vi "Bezier curve.vi"(2 "Segments":dbl, 3 "Parameters":cluster{"X":dbl, "Y":dbl}[](array[cluster])) -> (0 "XY Graph":cluster{dbl[], dbl[]}[](graph), 1 "Coordinate Array":cluster{"X":dbl, "Y":dbl}[](array[cluster]))   [LabVIEW 2020]
doc: "This VI uses the equation for a Bézier curve to create a set of coordinates."
panel:
  # "Test the Bezier curves"
  # "Formula:    B(t)  =  (1-t)^3 * P0 + 3 * (1-t)^2 * t * P1 + 3 * (1-t) * t^2 * P2 + t^3 * P3"
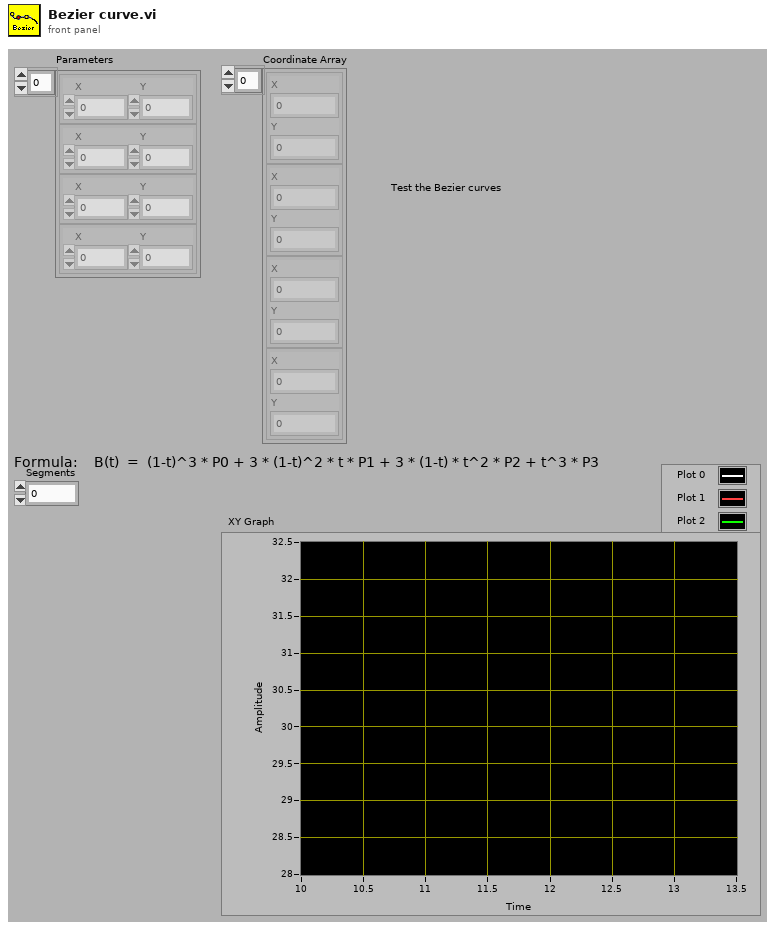
[diagram p1: front panel]
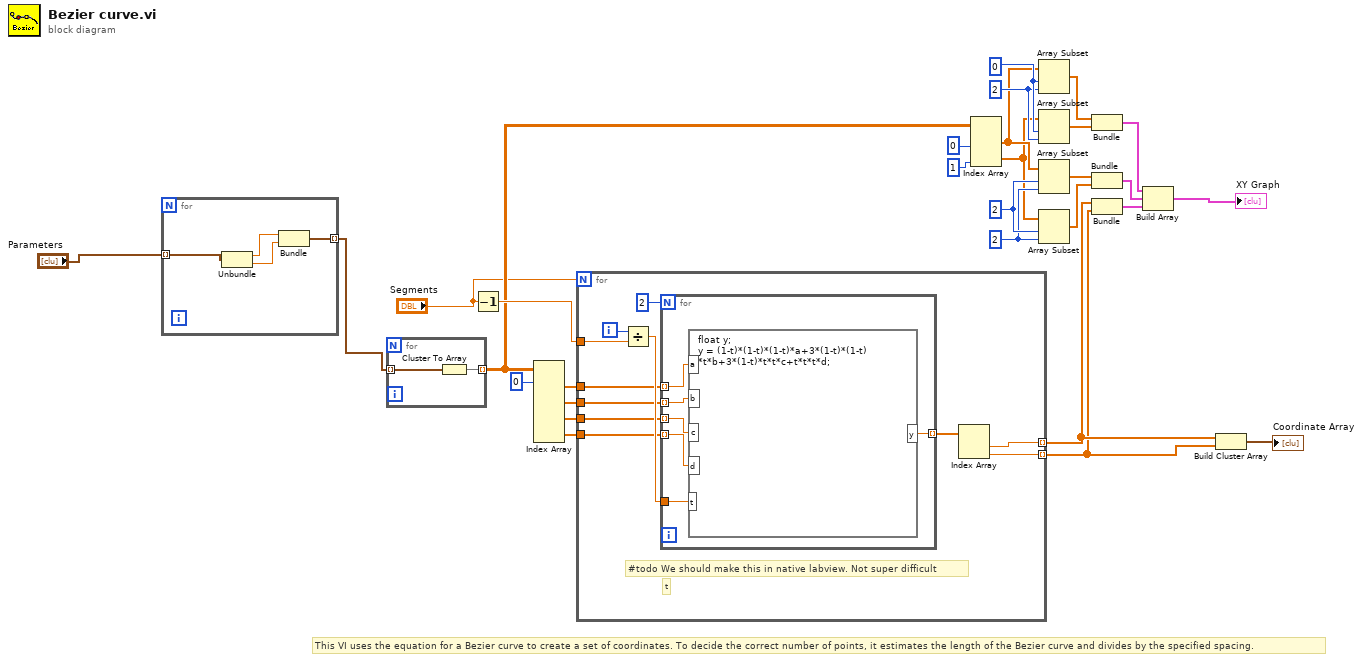
[diagram p0: block diagram]
diagram:
  w24 = 2 ("length")
  w25 = 2 ("index")
  w26 = 2 ("length")
  w27 = 0 ("index")
  # "This VI uses the equation for a Bezier curve to create a set of coordinates. To decide the correct number of points, it estimates the length of the Bezier curve and divides by the specified spacing."
  n1 = for {
    tunnel: "Parameters" -> [w33] mode=indexing
    tunnel: [w31] -> w3 mode=indexing
    n2 = Unbundle(w33) -> ("X"=w32:dbl, "Y"=w30:dbl)
    n3 = Bundle("X"=w32, "Y"=w30) -> (w31:cluster{"X":dbl, "Y":dbl})  [unwired: 1 in]
  }
  n4 = for {
    tunnel: w3 -> [w35] mode=indexing
    tunnel: [w34] -> w5 mode=indexing
    n5 = Cluster To Array(cluster=w35) -> (array=w34:dbl[])
  }
  n6 = Decrement(x="Segments") -> (x-1=w14:dbl)
  n7 = Index Array(array=w5, index (row) #1=0 ("index (row)")) -> (element #1=w12:dbl[], element #2=w11:dbl[], element #3=w10:dbl[], element #4=w9:dbl[])  [unwired: 7 in]
  n8 = for {
    N: "Segments" -> [_]
    tunnel: w12 -> [w43]
    tunnel: w14 -> [w45]
    tunnel: w11 -> [w42]
    tunnel: w10 -> [w41]
    tunnel: w9 -> [w40]
    tunnel: [w38] -> w7 mode=indexing
    tunnel: [w37] -> w2 mode=indexing
    i -> [w46]
    # "#todo We should make this in native labview. Not super difficult"
    # "t"
    n9 = Divide(x=w46, y=w45) -> (x/y=w44:dbl)
    n10 = for {
      N: 2 -> [_]
      tunnel: w44 -> [w52]
      tunnel: w43 -> [w51] mode=indexing
      tunnel: w42 -> [w50] mode=indexing
      tunnel: w41 -> [w49] mode=indexing
      tunnel: w40 -> [w48] mode=indexing
      tunnel: [w47] -> w39 mode=indexing
      n11 = formula code="float y;\ny = (1-t)*(1-t)*(1-t)*a+3*(1-t)*(1-t)\n*t*b+3*(1-t)*t*t*c+t*t*t*d;"("t"=w52, "a"=w51, "b"=w50, "c"=w49, "d"=w48) -> ("y"=w47:dbl)
    }
    n12 = Index Array(array=w39) -> (element #1=w38:dbl, element #2=w37:dbl)  [unwired: 2 in]
  }
  n13 = Index Array(array=w5, index (col) #1=0 ("disabled index (col)"), index (col) #2=1 ("index (col)")) -> (element #1=w23:dbl[], element #2=w8:dbl[])  [unwired: 2 in]
  n14 = Array Subset(array=w23, index=w27, length=w26) -> (w19:dbl[])
  n15 = Array Subset(array=w8, index=w27, length=w26) -> (w18:dbl[])
  n16 = Array Subset(array=w23, index=w25, length=w24) -> (w17:dbl[])
  n17 = Array Subset(array=w8, index=w25, length=w24) -> (w16:dbl[])
  n18 = Bundle(w19, w18) -> (w22:cluster{dbl[], dbl[]})  [unwired: 1 in]
  n19 = Bundle(w17, w16) -> (w21:cluster{dbl[], dbl[]})  [unwired: 1 in]
  n20 = Bundle(w7, w2) -> (w15:cluster{dbl[], dbl[]})  [unwired: 1 in]
  n21 = Build Array(w22, w21, w15) -> (→"XY Graph":cluster{dbl[], dbl[]}[])
  n22 = Build Cluster Array(w7, w2) -> (→"Coordinate Array":cluster{dbl, dbl}[])
